vi "Load App.vi"(8 "error in (no error)":errorcluster) -> (0 "error out":errorcluster)   [LabVIEW 2016]
uses:
  User Interface/User Interface.lvclass
  C:/Program Files (x86)/National Instruments/LabVIEW 2016/vi.lib/ActorFramework/Actor/Actor.lvclass
  <vilib>/ActorFramework/Actor/Actor.lvclass
  Configurations/Configurations.lvclass
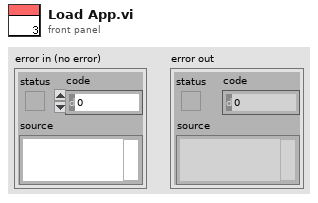
[diagram p1: front panel]
types:
  T1 = typedef "Configurations.lvlib/Configurations.lvclass/Session Handle.ctl" = refnum<data-value>
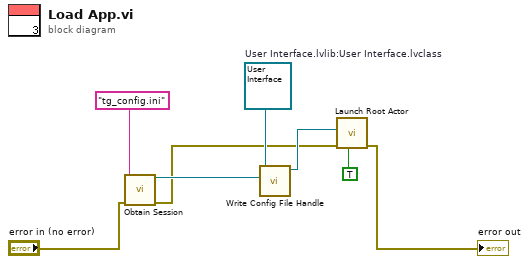
[diagram p0: block diagram]
diagram:
  w3 = refnum<class "User Interface.lvclass"> refnum  # User Interface.lvlib:User Interface.lvclass
  n1 = call "Obtain Session.vi"("Filename"="tg_config.ini", "error in (no error)"="error in (no error)") -> ("Session Handle"=w6:T1, "error out"=w1:errorcluster)  [unwired: 12 in]
  n2 = call-dynamic "Write Config File Handle.vi"("Session Handle"=w6, "User Interface in"=w3) -> ("User Interface out"=w4:refnum<class "User Interface.lvclass">)  [unwired: 9 in]
  n3 = call <vilib>:"Launch Root Actor.vi"("Open Actor Core front panel? (F)"=TRUE, "error in (no error)"=w1, "Actor"=w4) -> ("error out"=→"error out":errorcluster)  [unwired: 7 in, 1 out]
